vi "Get Status.vi"(8 "error in (no error)":errorcluster, 11 "Filter Wheel Simulator in":refnum<class "Filter Wheel Simulator.lvclass">) -> (0 "error out":errorcluster, 2 "FW Status":T1={"State"=enum."Move Complete", "Positions"=[], "Names"=[], "Notch"=[], "Moving"=[FALSE, FALSE]}, 3 "Filter Wheel Simulator out":refnum<class "Filter Wheel Simulator.lvclass">)   [LabVIEW 2021, in "Filter Wheel Simulator.lvclass"]
uses:
  Filter Wheel Simulator.lvclass
  C:/Development/prime/Prime-RIMAS/Filter Wheel/Filter Wheel Object/Filter Wheel.lvclass
  FW cluster Status.ctl
  FW enum status.ctl
  Filter Wheel Object/Filter Wheel.lvclass
  Filter Wheel Simulator.lvclass/Filter Wheel Simulator.ctl
  Filter Wheel Object/Filter Wheel.lvclass/Filter Wheel.ctl
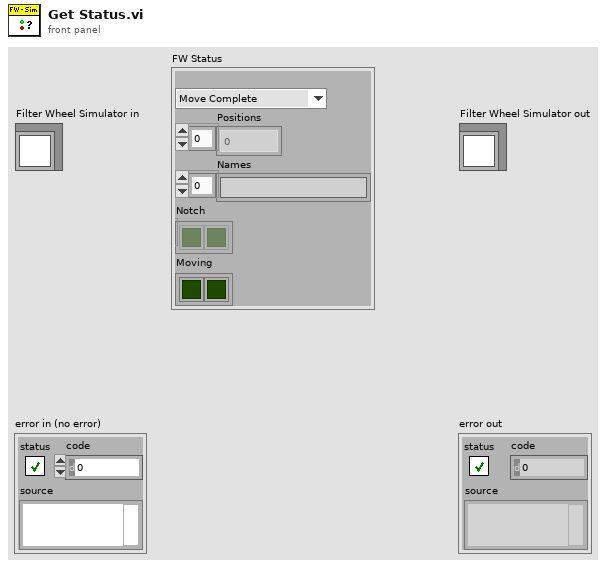
[diagram p1: front panel]
types:
  T1 = typedef "FW cluster Status.ctl" = cluster{"State":T2, "Positions":i32[], "Names":string[], "Notch":bool[], "Moving":bool[]}
  T2 = typedef "FW enum status.ctl" = enum16{"Initializing", "Moving", "Move Complete", "Error"}
  T3 = typedef "Filter Wheel Simulator.lvclass/Filter Wheel cluster Simulated Status.ctl" = cluster{"Move Start Time":timestamp, "Moving?":bool, "Target Pos":dbl, "Direction":bool}
  T4 = typedef "Filter Wheel Simulator.lvclass/Filter Wheel Move cluster.ctl" = cluster{"Wheel":i32, "Target Pos":i32}
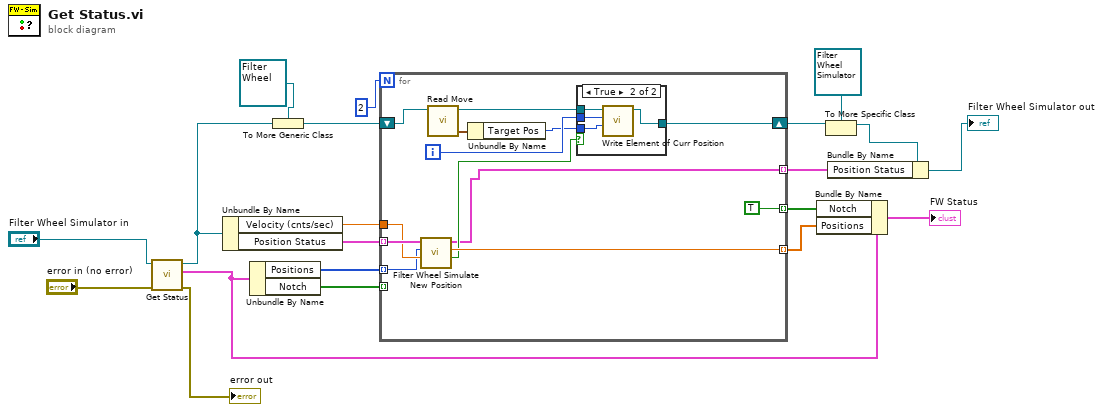
[diagram p0: block diagram]
diagram:
  n1 = call-parent "Get Status.vi"("error in (no error)"="error in (no error)", "Filter Wheel in"="Filter Wheel Simulator in") -> ("error out"=→"error out":errorcluster, "FW Status"=w14:T1, "Filter Wheel out"=w8:refnum<class "Filter Wheel Simulator.lvclass">)  [unwired: 7 in]
  n2 = Unbundle By Name(w8) -> ("Velocity (cnts/sec)"=w17:dbl, "Position Status"=w18:T3[])
  n3 = Unbundle By Name(w14) -> ("Positions"=w16:i32[], "Notch"=w15:bool[])
  n4 = To More Generic Class(target class=refnum<class "Filter Wheel.lvclass"> refnum ("Filter Wheel.lvclass"), reference=w8) -> (generic class reference=w6:refnum<class "Filter Wheel.lvclass">)
  n5 = for {
    N: 2 -> [_]
    tunnel: w18 -> [w33] mode=indexing
    tunnel: w17 -> [w32]
    tunnel: w16 -> [w31] mode=indexing
    tunnel: w15 -> [_] mode=indexing
    tunnel: [TRUE] -> w13 mode=indexing
    tunnel: [w30] -> w12 mode=indexing
    shift-right: [w23] -> w5
    shift-left: w6 -> [w28]
    tunnel: [w22] -> w2 mode=indexing
    i -> [w29]
    n6 = call "Filter Wheel Simulate New Position.vi"("Velocity (cnts/sec)"=w32, "Position"=w31, "Axis Status"=w33) -> ("move complete"=w25:bool, "New Pos"=w30:dbl, "Axis Status Out"=w22:T3)  [unwired: 6 in]
    n7 = call "Read Move.vi"("Filter Wheel in"=w28) -> ("Move"=w27:T4, "Filter Wheel out"=w26:refnum<class "Filter Wheel.lvclass">)  [unwired: 8 in, 1 out]
    n8 = Unbundle By Name(w27) -> ("Target Pos"=w24:i32)
    n9 = case shown="True" w25 {
      tunnel: w29 -> [_ w38]
      tunnel: w26 -> [w34 w37]
      tunnel: [w34 w36] -> w23
      tunnel: w24 -> [_ w35]
      frame False {
      }
      frame True {
        n10 = call "Write Element of Curr Position.vi"("Position idx"=w35, "Wheel"=w38, "Filter Wheel in"=w37) -> ("Filter Wheel out"=w36:refnum<class "Filter Wheel.lvclass">)  [unwired: 7 in, 1 out]
      }
    }
  }
  n11 = Bundle By Name(cluster=w14, "Notch"=w13, "Positions"=w12) -> (→"FW Status":T1)
  n12 = To More Specific Class(target class=refnum<class "Filter Wheel Simulator.lvclass"> refnum ("Filter Wheel Simulator out"), reference=w5) -> (specific class reference=w3:refnum<class "Filter Wheel Simulator.lvclass">)  [unwired: 1 in, 1 out]
  n13 = Bundle By Name(cluster=w3, "Position Status"=w2) -> (→"Filter Wheel Simulator out":refnum<class "Filter Wheel Simulator.lvclass">)
